vi "Download Files.vi"(8 "error in (no error)":errorcluster, 11 "Item Ref in":T1 format="%.0x") -> (0 "error out":errorcluster, 1 "mmanager":path, 2 "vclient":path, 3 "Device Ref out":T1 format="%.0x")   [LabVIEW 2020, in "Vires VTD System Explorer.lvlib"]
uses:
  Vires VTD System Explorer.lvlib
  <vilib>/NI VeriStand/Custom Device API/Custom Device Item Ref.ctl
  <vilib>/NI VeriStand/Custom Device API/Custom Device File Dependency.ctl
  <vilib>/NI VeriStand/Custom Device API/Path Specification.ctl
  <vilib>/NI VeriStand/Custom Device API/Path Type.ctl
  <vilib>/NI VeriStand/Custom Device API/Custom Device Supported Target.ctl
  <vilib>/NI VeriStand/Custom Device API/Custom Device API.lvlib
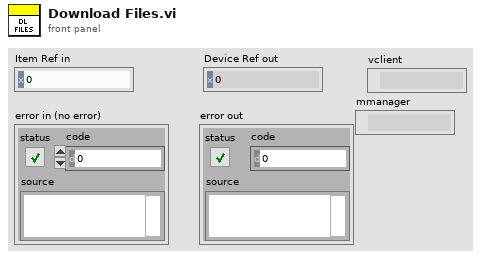
[diagram p1: front panel]
types:
  T1 = typedef "Custom Device API.lvlib/Custom Device Item Ref.ctl" = u64
  T2 = typedef "Custom Device API.lvlib/Custom Device Target Type.ctl" = enum16{"PharLap", "VxWorks", "Windows", "Linux_32_ARM", "Linux_x64"}
  T3 = typedef "Custom Device API.lvlib/Custom Device File Dependency.ctl" = cluster{"Source":T4, "RT Destination":path, "ForceDownload?":bool, "SupportedTarget":T6, "Version":string}
  T4 = typedef "Custom Device API.lvlib/Path Specification.ctl" = cluster{"Path":path, "Type":T5}
  T5 = typedef "Custom Device API.lvlib/Path Type.ctl" = enum16{"Absolute", "To Base", "To Common Data Dir", "To Application Data Dir"}
  T6 = typedef "Custom Device API.lvlib/Custom Device Supported Target.ctl" = enum16{"All", "PharLap", "VxWorks", "Windows", "Linux_32_ARM", "Linux_x64", "PharLap & Windows", "PharLap & VxWorks", "VxWorks & Windows"}
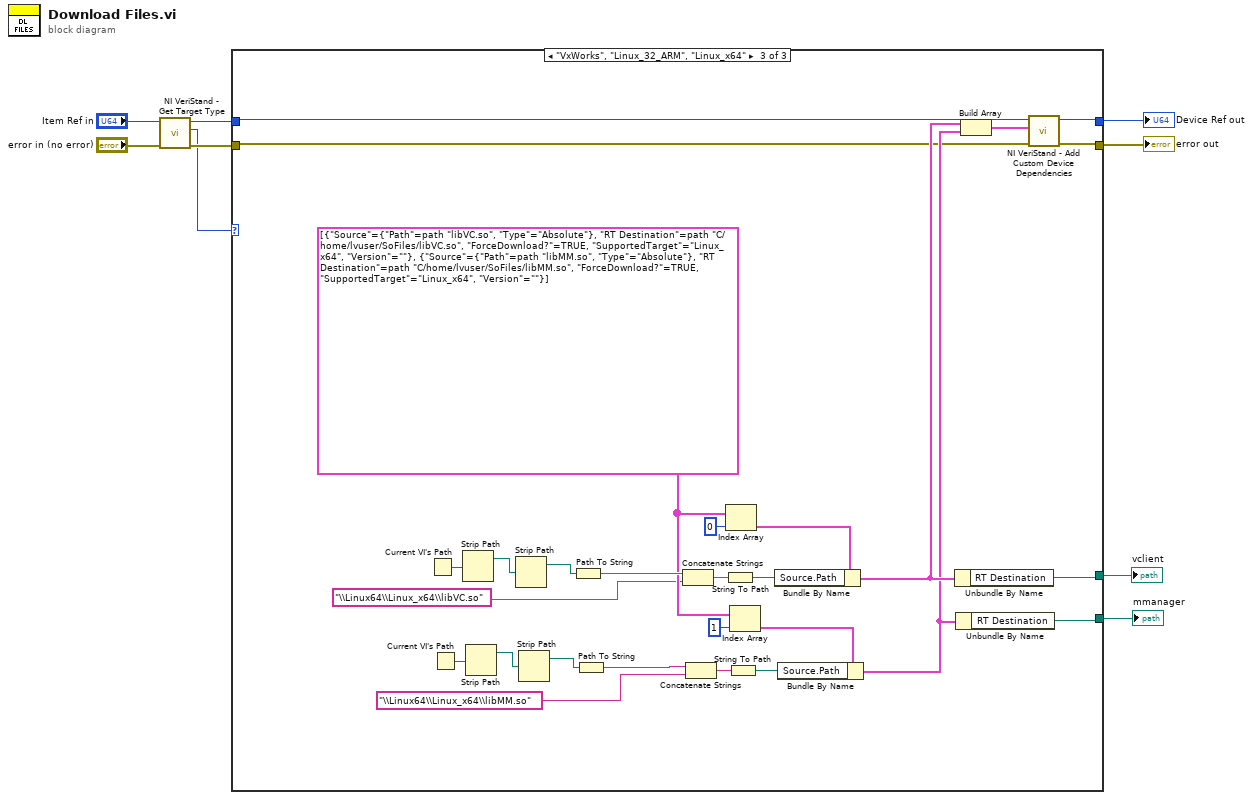
[diagram p0: block diagram]
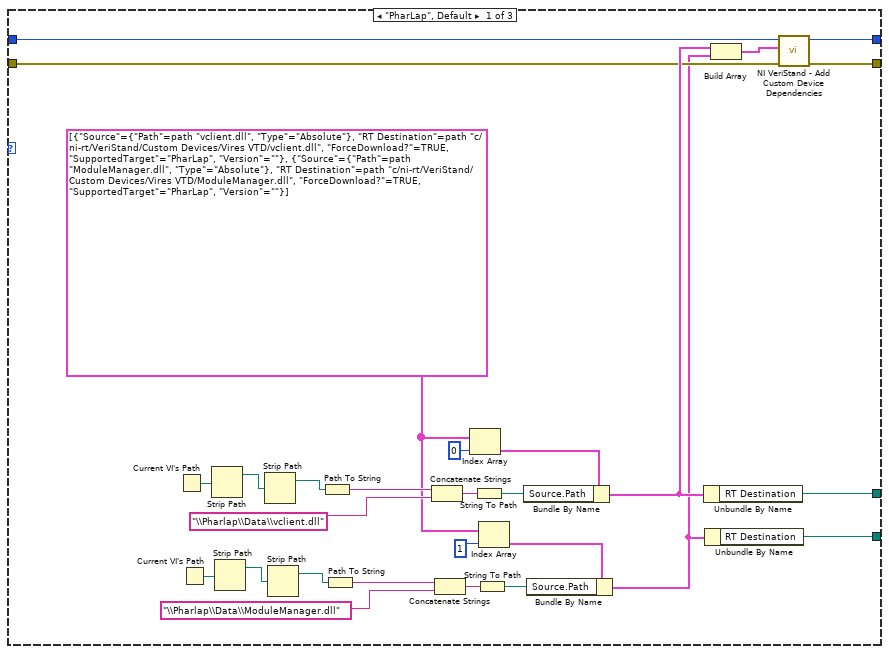
[diagram p2: hidden frame]
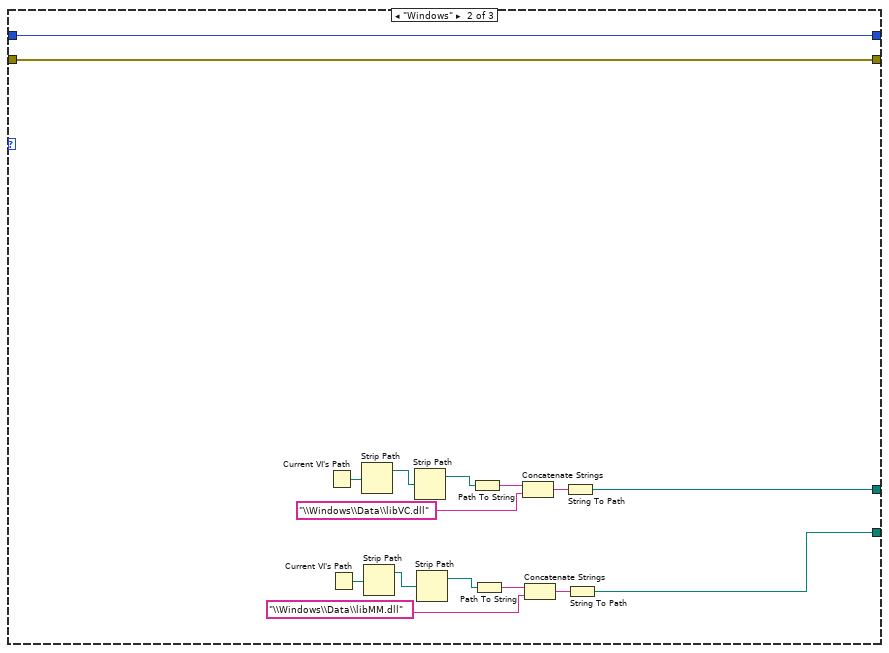
[diagram p3: hidden frame]
diagram:
  n1 = call <vilib>:"NI VeriStand - Get Target Type.vi"("error in (no error)"="error in (no error)", "Item Ref in"="Item Ref in") -> ("error out"=w6:errorcluster, "Target Type"=w5:T2, "Item Ref out"=w8:T1)  [unwired: 7 in]
  n2 = case shown="\"VxWorks\", \"Linux_32_ARM\", \"Linux_x64\"" w5 {
    tunnel: [w30 w52 w58] -> w4
    tunnel: w8 -> [w25 w53 w60]
    tunnel: w6 -> [w24 w52 w61]
    tunnel: [w29 w53 w59] -> w3
    tunnel: [w26 w39 w57] -> w2
    tunnel: [w13 w38 w56] -> w1
    frame "PharLap", Default {
      w16 = T3[] [{"Source"={"Path"=path "vclient.dll", "Type"=enum."Absolute"}, "RT Destination"=path "c:/ni-rt/VeriStand/Custom Devices/Vires VTD/vclient.dll", "ForceDownload?"=TRUE, "SupportedTarget"=enum."PharLap", "Version"=""}, {"Source"={"Path"=path "ModuleManager.dll", "Type"=enum."Absolute"}, "RT Destination"=path "c:/ni-rt/VeriStand/Custom Devices/Vires VTD/ModuleManager.dll", "ForceDownload?"=TRUE, "SupportedTarget"=enum."PharLap", "Version"=""}] ("Dependencies")
      n3 = Current VI's Path() -> (path=w32:path)
      n4 = Current VI's Path() -> (path=w22:path)
      n5 = Strip Path(path=w32) -> (stripped path=w33:path)  [unwired: 1 out]
      n6 = Strip Path(path=w22) -> (stripped path=w21:path)  [unwired: 1 out]
      n7 = Strip Path(path=w33) -> (stripped path=w34:path)  [unwired: 1 out]
      n8 = Strip Path(path=w21) -> (stripped path=w20:path)  [unwired: 1 out]
      n9 = Path To String(path=w34) -> (string=w35:string)
      n10 = Path To String(path=w20) -> (string=w19:string)
      n11 = Concatenate Strings(w35, "\\Pharlap\\Data\\vclient.dll" ("name or relative path")) -> (w11:string)
      n12 = Concatenate Strings(w19, "\\Pharlap\\Data\\ModuleManager.dll" ("name or relative path")) -> (w10:string)
      n13 = Index Array(array=w16, index=0) -> (element=w37:T3)
      n14 = String To Path(string=w11) -> (path=w31:path)
      n15 = String To Path(string=w10) -> (path=w23:path)
      n16 = Index Array(array=w16, index=1) -> (element=w17:T3)
      n17 = Bundle By Name(cluster=w37, "Source.Path"=w31) -> (w27:T3)
      n18 = Bundle By Name(cluster=w17, "Source.Path"=w23) -> (w12:T3)
      n19 = Unbundle By Name(w27) -> ("RT Destination"=w26:path)
      n20 = Unbundle By Name(w12) -> ("RT Destination"=w13:path)
      n21 = Build Array(w27, w12) -> (w28:T3[])
      n22 = call <vilib>:"NI VeriStand - Add Custom Device Dependencies.vi"("error in (no error)"=w24, "Dependencies"=w28, "Device Ref in"=w25) -> ("error out"=w30:errorcluster, "Device Ref out"=w29:T1)  [unwired: 7 in]
    }
    frame "Windows" {
      n23 = Current VI's Path() -> (path=w46:path)
      n24 = Current VI's Path() -> (path=w45:path)
      n25 = Strip Path(path=w46) -> (stripped path=w47:path)  [unwired: 1 out]
      n26 = Strip Path(path=w45) -> (stripped path=w40:path)  [unwired: 1 out]
      n27 = Strip Path(path=w47) -> (stripped path=w48:path)  [unwired: 1 out]
      n28 = Strip Path(path=w40) -> (stripped path=w44:path)  [unwired: 1 out]
      n29 = Path To String(path=w48) -> (string=w49:string)
      n30 = Path To String(path=w44) -> (string=w43:string)
      n31 = Concatenate Strings(w49, "\\Windows\\Data\\libVC.dll" ("name or relative path")) -> (w51:string)
      n32 = Concatenate Strings(w43, "\\Windows\\Data\\libMM.dll" ("name or relative path")) -> (w41:string)
      n33 = String To Path(string=w51) -> (path=w39:path)
      n34 = String To Path(string=w41) -> (path=w38:path)
    }
    frame "VxWorks", "Linux_32_ARM", "Linux_x64" {
      w67 = T3[] [{"Source"={"Path"=path "libVC.so", "Type"=enum."Absolute"}, "RT Destination"=path "C:/home/lvuser/SoFiles/libVC.so", "ForceDownload?"=TRUE, "SupportedTarget"=enum."Linux_x64", "Version"=""}, {"Source"={"Path"=path "libMM.so", "Type"=enum."Absolute"}, "RT Destination"=path "C:/home/lvuser/SoFiles/libMM.so", "ForceDownload?"=TRUE, "SupportedTarget"=enum."Linux_x64", "Version"=""}] ("Dependencies")
      n35 = Current VI's Path() -> (path=w77:path)
      n36 = Current VI's Path() -> (path=w72:path)
      n37 = Strip Path(path=w77) -> (stripped path=w78:path)  [unwired: 1 out]
      n38 = Strip Path(path=w72) -> (stripped path=w71:path)  [unwired: 1 out]
      n39 = Strip Path(path=w78) -> (stripped path=w79:path)  [unwired: 1 out]
      n40 = Strip Path(path=w71) -> (stripped path=w70:path)  [unwired: 1 out]
      n41 = Path To String(path=w79) -> (string=w80:string)
      n42 = Path To String(path=w70) -> (string=w69:string)
      n43 = Concatenate Strings(w80, "\\Linux64\\Linux_x64\\libVC.so" ("name or relative path")) -> (w63:string)
      n44 = Concatenate Strings(w69, "\\Linux64\\Linux_x64\\libMM.so" ("name or relative path")) -> (w62:string)
      n45 = String To Path(string=w63) -> (path=w76:path)
      n46 = Index Array(array=w67, index=0) -> (element=w81:T3)
      n47 = String To Path(string=w62) -> (path=w73:path)
      n48 = Index Array(array=w67, index=1) -> (element=w68:T3)
      n49 = Bundle By Name(cluster=w81, "Source.Path"=w76) -> (w74:T3)
      n50 = Bundle By Name(cluster=w68, "Source.Path"=w73) -> (w64:T3)
      n51 = Unbundle By Name(w74) -> ("RT Destination"=w57:path)
      n52 = Unbundle By Name(w64) -> ("RT Destination"=w56:path)
      n53 = Build Array(w74, w64) -> (w75:T3[])
      n54 = call <vilib>:"NI VeriStand - Add Custom Device Dependencies.vi"("error in (no error)"=w61, "Dependencies"=w75, "Device Ref in"=w60) -> ("error out"=w58:errorcluster, "Device Ref out"=w59:T1)  [unwired: 7 in]
    }
  }
  "error out" <- w4
  "Device Ref out" <- w3
  "vclient" <- w2
  "mmanager" <- w1
